vi "CAN Queue Ref FGV.vi"(6 "CAN FGV State":T2=enum."Get", 8 "error in":errorcluster, 11 "CAN Read Q In":T1) -> (0 "error out":errorcluster, 3 "CAN Read Q Out":T1)   [LabVIEW 2023, in "LTT_TeststandSteptypes.lvlib"]
uses:
  LTT_TeststandSteptypes.lvlib
  Control/CAN Read Q Ref.ctl
  <vilib>/xnet/xnet.llb/XNET Frame CAN.ctl
  <vilib>/xnet/xnet.llb/XNET Frame Type CAN.ctl
  Control/CAN FGV State.ctl
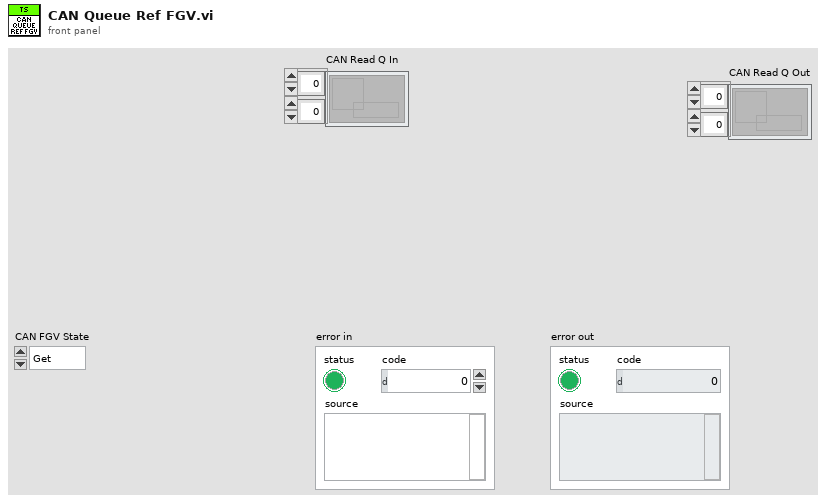
[diagram p1: front panel]
types:
  T1 = typedef "LTT_TeststandSteptypes.lvlib/CAN Read Q Ref.ctl" = refnum<queue>[][]
  T2 = typedef "LTT_TeststandSteptypes.lvlib/CAN FGV State.ctl" = enum16{"Init", "Get", "Set"}
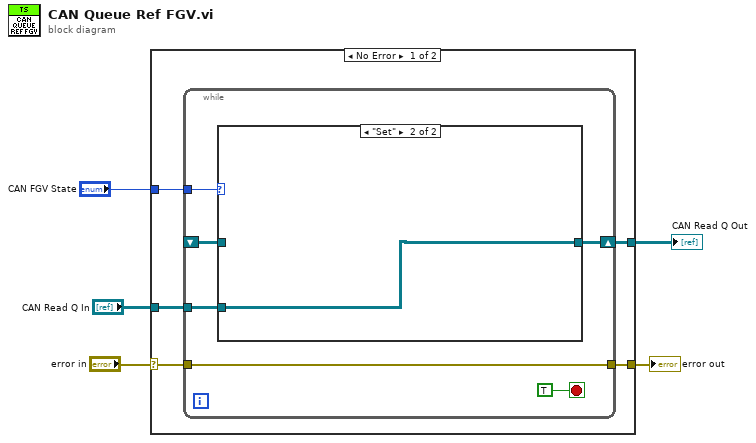
[diagram p0: block diagram]
diagram:
  n1 = case shown="No Error" "error in" {
    selector: "error in" -> [w10 w19]
    tunnel: "CAN FGV State" -> [w9 _]
    tunnel: [w8 w19] -> w3
    tunnel: "CAN Read Q In" -> [w7 _]
    tunnel: [w6 _] -> w1
    frame No Error {
      n2 = while {
        tunnel: w10 -> [w12]
        tunnel: w9 -> [w15]
        shift-right: [w14] -> w6
        shift-left: _ -> [w13]
        tunnel: [w12] -> w8
        tunnel: w7 -> [w11]
        stop <- TRUE stop-if-true
        n3 = case shown="\"Set\"" w15 {
          tunnel: [w17 w18] -> w14
          tunnel: w13 -> [w17 _]
          tunnel: w11 -> [_ w18]
          frame "Get", Default {
          }
          frame "Set" {
          }
        }
      }
    }
    frame Error {
    }
  }
  "error out" <- w3
  "CAN Read Q Out" <- w1
